vi "Test VIPM Update Job.vi"() -> ()   [LabVIEW 2014]
uses:
  Core/LabVIEW CI Service/Extensions/VIPM Update/VIPM Update/VIPM Update - STYP.ctl
  Core/LabVIEW CI Service/Classes/Status Updater/Status Updater.lvclass/Status Updater.ctl
  Core/LabVIEW CI Service/Classes/Job/Job.lvclass/Job.ctl
  Core/LabVIEW CI Service/Extensions/VIPM Update/VIPM Update/VIPM Update.lvclass
  Core/LabVIEW CI Service/Classes/Status Updater/Status Updater.lvclass
  Core/LabVIEW CI Service/Classes/Job/Job.lvclass
panel:
  in  "LabVIEW Version":string="14.0"
  in  "Workspace Path":path=path "P:/alsmith/Sales/users/ACS/LabVIEW Continuous Integration/Jenkins Sample Project/Run VI Golden DUT.vi"
  out "Results":T1 {"Status" items=["Service Error"=504, "Abort"=503, "Fail"=500, "Pass"=200]}
  out "Steps":string[](array[string])
  out "Progress Percents":u32[](array[numeric])
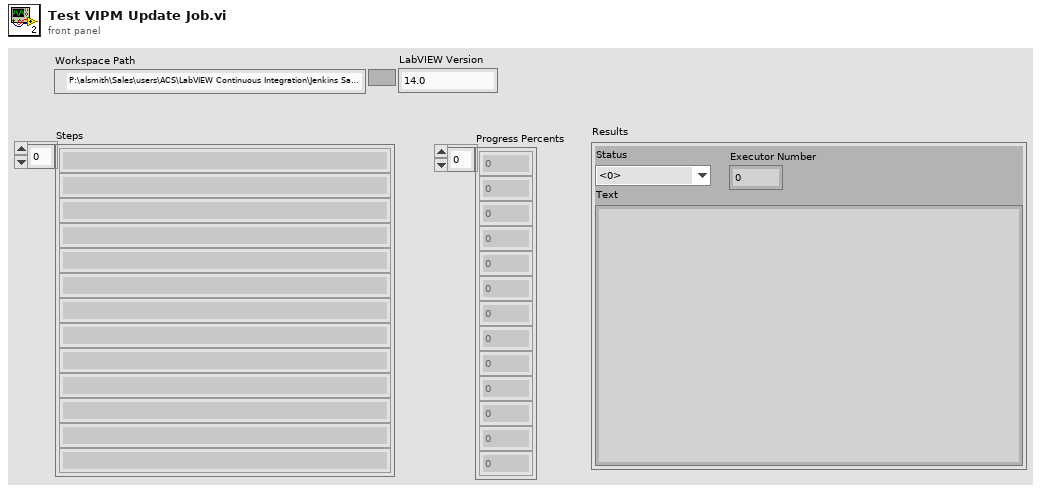
[diagram p1: front panel]
types:
  T1 = cluster{"Status":u16, "Text":string, "Executor Number":i32}
  T2 = typedef "VIPM Update - STYP.ctl" = cluster{"LabVIEW Version":string}
  T3 = cluster{"Event Registration Refnum":refnum<event-registration>, "Event Registration Refnum":refnum<event-registration>}
  T4 = typedef "Job Results - STYP.ctl" = cluster{"Status":u16, "Text":string, "Executor Number":i32}
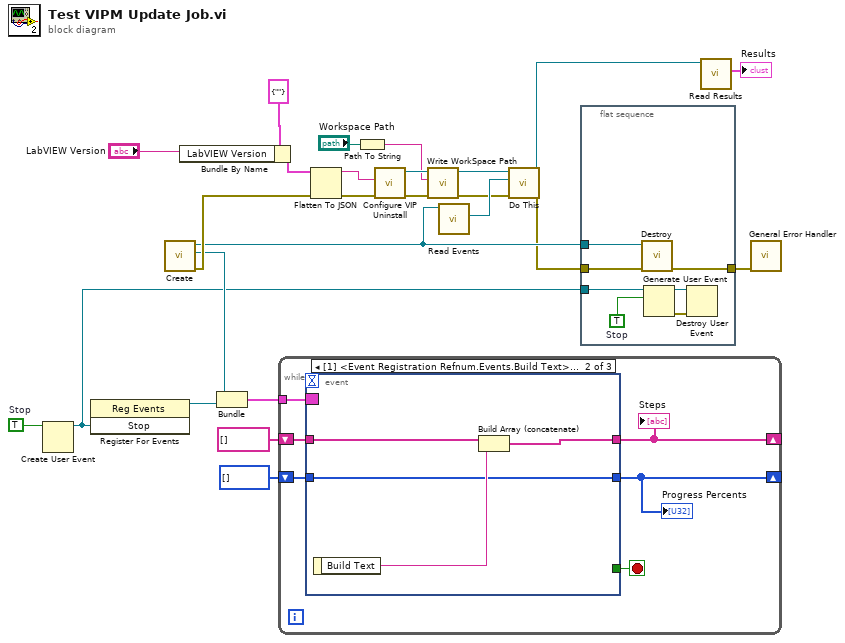
[diagram p0: block diagram]
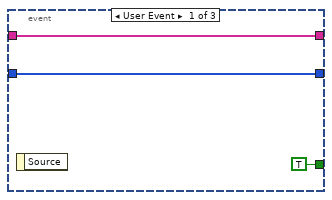
[diagram p2: hidden frame]
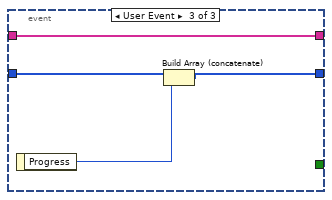
[diagram p3: hidden frame]
diagram:
  w23 = TRUE  # Stop
  n1 = Create User Event(user event datatype=w23) -> (user event=w19:refnum<user-event>)  [unwired: 1 in, 1 out]
  n2 = register-events(w19) -> (reference out=w20:refnum<event-registration>)  [unwired: 2 in, 1 out]
  n3 = call "Create.vi"() -> ("error out"=w24:errorcluster, "Event Registration Refnum"=w22:refnum<event-registration>, "Status Updater out"=w14:refnum<class "Status Updater.lvclass">)  [unwired: 9 in]
  n4 = Bundle By Name(cluster=T2 {"LabVIEW Version"=""} ("VIPM Update"), "LabVIEW Version"="LabVIEW Version") -> (w25:T2)
  n5 = Bundle("Event Registration Refnum"=w22, "Event Registration Refnum"=w20) -> (w21:T3)  [unwired: 1 in]
  n6 = while {
    tunnel: w21 -> [w31]
    shift-right: [w27] -> _
    shift-left: string[] [] -> [w29]
    shift-right: [w26] -> _
    shift-left: u32[] [] -> [w28]
    stop <- w30 stop-if-true
    n7 = event shown="[1] <Event Registration Refnum.Events.Build Text>: User Event" {
      selector: w31 -> [_ _ _]
      dyn-events: _ -> [_ _ _]
      timeout: _ -> [_ _ _]
      tunnel: [TRUE _ _] -> w30
      tunnel: w29 -> [w33 w38 w42]
      tunnel: [w33 w37 w42] -> w27
      tunnel: w28 -> [w32 w35 w41]
      tunnel: [w32 w35 w40] -> w26
      event User Event {
        n8 = event-data() -> ()  [unwired: 1 in, 1 out]
      }
      event User Event {
        n9 = event-data() -> ("Build Text"=w36:string)  [unwired: 1 in]
        n10 = Build Array (concatenate)(w38, w36) -> (w37:string[])
      }
      event User Event {
        n11 = event-data() -> ("Progress"=w39:u32)  [unwired: 1 in]
        n12 = Build Array (concatenate)(w41, w39) -> (w40:u32[])
      }
    }
    "Steps" <- w27
    "Progress Percents" <- w26
  }
  n13 = Flatten To JSON(anything=w25, error in (no error)=w24) -> (JSON string=w12:string, 11:w13:errorcluster)  [unwired: 1 in]
  n14 = Path To String(path="Workspace Path") -> (string=w4:string)
  n15 = call "Configure VIP Uninstall.vi"("error in (no error)"=w13, "JSON string"=w12) -> ("error out"=w5:errorcluster, "VIP Install Out"=w6:refnum<class "VIPM Update.lvclass">)  [unwired: 8 in]
  n16 = call "Write WorkSpace Path.vi"("error in (no error)"=w5, "WorkSpace Path"=w4, "Job in"=w6) -> ("error out"=w2:errorcluster, "Job out"=w3:refnum<class "VIPM Update.lvclass">)  [unwired: 7 in]
  n17 = call "Read Events.vi"("Status Updater in"=w14) -> ("Status Events"=w10:refnum<class "Status Events.lvclass">)  [unwired: 10 in]
  n18 = call-dynamic "Do This.vi"("error in (no error)"=w2, "Status Events"=w10, "VIP Uninstall in"=w3) -> ("error out"=w8:errorcluster, "VIP Uninstall out"=w9:refnum<class "VIPM Update.lvclass">)  [unwired: 7 in]
  n19 = flat-sequence {
    tunnel: w14 -> [w49]
    tunnel: w8 -> [w48]
    tunnel: w19 -> [w46]
    tunnel: [w45] -> w16
    frame #0 {
      w47 = TRUE  # Stop
      n20 = call "Destroy.vi"("error in (no error)"=w48, "Status Updater in"=w49) -> ("error out"=w45:errorcluster)  [unwired: 9 in]
      n21 = Generate User Event(user event=w46, event data cluster=w47) -> (user event out=w43:refnum<user-event>, error out=w44:errorcluster)  [unwired: 2 in]
      n22 = Destroy User Event(user event=w43, error in=w44) -> ()  [unwired: 1 out]
    }
  }
  n23 = call "Read Results.vi"("Job in"=w9) -> ("Results"=→"Results":T4)  [unwired: 10 in]
  n24 = call <vilib>:"General Error Handler.vi"("error in (no error)"=w16) -> ()  [unwired: 10 in, 5 out]
